vi "update.vi"(0 "OWEN HMI.lvclass":refnum<class "OWEN HMI.lvclass">, 11 "error in":errorcluster) -> (15 "error out":errorcluster)   [LabVIEW 2019, in "OWEN HMI.lvclass"]
uses:
  OWEN HMI.lvclass
  Bit.ctl
  Words.ctl
  19f3744f-72bc-4c39-aaca-5bdf827a74e4.vi
  b80abefe-0104-4203-839a-19dc6cb4a819.vi
  Global - Data.vi
panel:
  in  "stop":bool
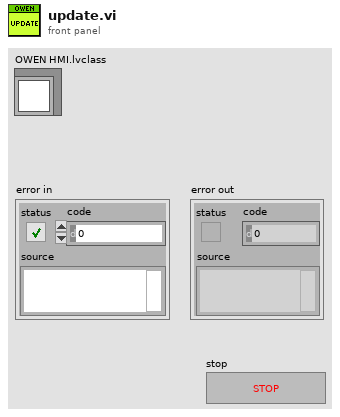
[diagram p1: front panel]
types:
  T1 = typedef "OWEN HMI.lvclass/Bit.ctl" = enum16{"0 - Pump CC", "1 - Pump SO", "2 - Alarm", "3 - Warning", "4 - DUT", "5 - CHMBR"}
  T2 = typedef "OWEN HMI.lvclass/Words.ctl" = enum16{"0 - Bits", "1 - Level CC", "2 - Temp CC", "3 - Level SO", "4 - Temp SO"}
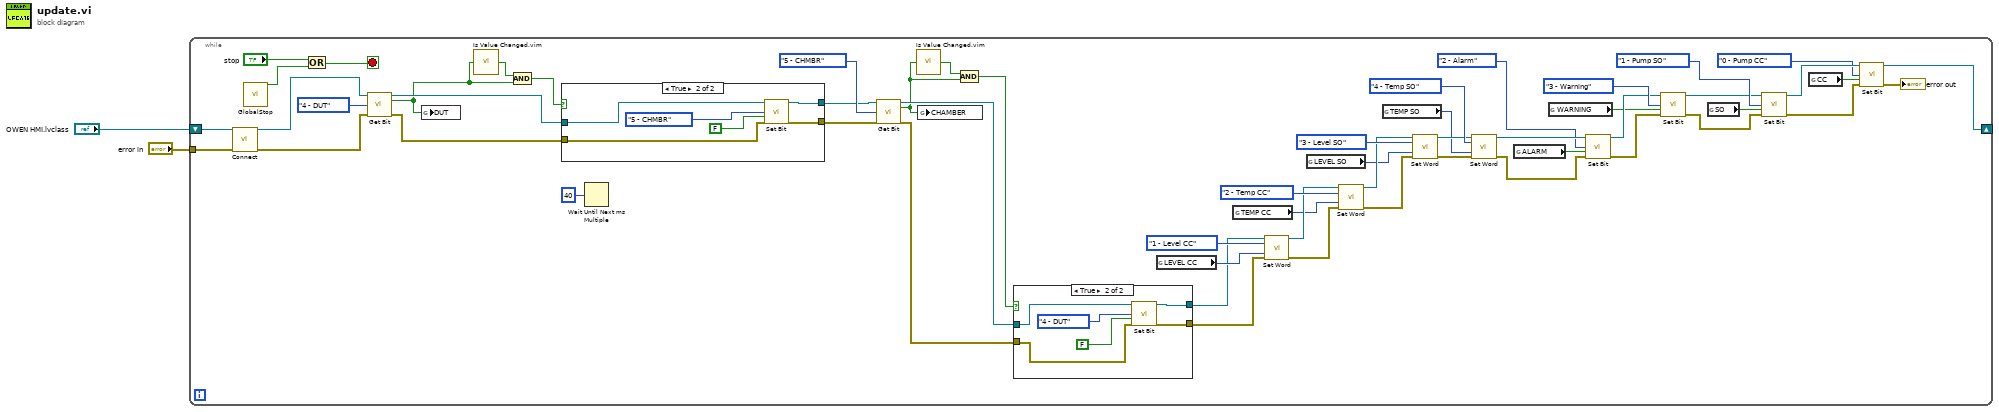
[diagram p0: block diagram]
diagram:
  n1 = while {
    tunnel: "error in" -> [w58]
    shift-right: [w6] -> _
    shift-left: "OWEN HMI.lvclass" -> [w30]
    stop <- w4 stop-if-true
    n2 = call "Connect.vi"("OWEN HMI in"=w30, "error in (no error)"=w58) -> ("OWEN HMI out"=w57:refnum<class "OWEN HMI.lvclass">, "error out"=w56:errorcluster)  [unwired: 12 in]
    n3 = call "GlobalStop.vi"() -> ("Stop"=w3:bool)  [unwired: 15 in]
    n4 = Or(x="stop", y=w3) -> (x .or. y?=w4:bool)
    n5 = call "Get Bit.vi"("OWEN HMI in"=w57, "bit"=Bit."4 - DUT", "error in (no error)"=w56) -> ("OWEN HMI out"=w55:refnum<class "OWEN HMI.lvclass">, "value"=w22:bool, "error out"=w54:errorcluster)  [unwired: 10 in]
    n6 = global write "Global - Data.vi" "DUT"(w22) -> ()
    n7 = call "Is Value Changed.vim"("value"=w22) -> ("changed or first call?"=w21:bool)
    n8 = And(x=w21, y=w22) -> (x .and. y?=w52:bool)
    n9 = case shown="True" w52 {
      tunnel: w55 -> [w68 w74]
      tunnel: w54 -> [w67 w73]
      tunnel: [w68 w71] -> w20
      tunnel: [w67 w70] -> w19
      frame False {
      }
      frame True {
        n10 = call "Set Bit.vi"("OWEN HMI in"=w74, "bit"=Bit."5 - CHMBR", "value"=FALSE, "error in (no error)"=w73) -> ("OWEN HMI out"=w71:refnum<class "OWEN HMI.lvclass">, "error out"=w70:errorcluster)  [unwired: 10 in]
      }
    }
    n11 = Wait Until Next ms Multiple(millisecond multiple=u32 40 ("milliseconds to wait")) -> ()  [unwired: 1 out]
    n12 = call "Get Bit.vi"("OWEN HMI in"=w20, "bit"=Bit."5 - CHMBR", "error in (no error)"=w19) -> ("OWEN HMI out"=w49:refnum<class "OWEN HMI.lvclass">, "value"=w16:bool, "error out"=w50:errorcluster)  [unwired: 10 in]
    n13 = call "Is Value Changed.vim"("value"=w16) -> ("changed or first call?"=w17:bool)
    n14 = global write "Global - Data.vi" "CHAMBER"(w16) -> ()
    n15 = And(x=w17, y=w16) -> (x .and. y?=w51:bool)
    n16 = case shown="True" w51 {
      tunnel: w49 -> [w60 w66]
      tunnel: w50 -> [w59 w65]
      tunnel: [w60 w63] -> w18
      tunnel: [w59 w62] -> w15
      frame False {
      }
      frame True {
        n17 = call "Set Bit.vi"("OWEN HMI in"=w66, "bit"=Bit."4 - DUT", "value"=FALSE, "error in (no error)"=w65) -> ("OWEN HMI out"=w63:refnum<class "OWEN HMI.lvclass">, "error out"=w62:errorcluster)  [unwired: 10 in]
      }
    }
    n18 = global read "Global - Data.vi" "LEVEL CC"() -> (w24:i16)
    n19 = global read "Global - Data.vi" "TEMP CC"() -> (w25:i16)
    n20 = call "Set Word.vi"("OWEN HMI in"=w18, "address"=Words."1 - Level CC", "value"=w24, "error in (no error)"=w15) -> ("OWEN HMI out"=w46:refnum<class "OWEN HMI.lvclass">, "error out"=w45:errorcluster)  [unwired: 10 in]
    n21 = global read "Global - Data.vi" "LEVEL SO"() -> (w26:i16)
    n22 = call "Set Word.vi"("OWEN HMI in"=w46, "address"=Words."2 - Temp CC", "value"=w25, "error in (no error)"=w45) -> ("OWEN HMI out"=w43:refnum<class "OWEN HMI.lvclass">, "error out"=w42:errorcluster)  [unwired: 10 in]
    n23 = global read "Global - Data.vi" "TEMP SO"() -> (w27:i16)
    n24 = call "Set Word.vi"("OWEN HMI in"=w43, "address"=Words."3 - Level SO", "value"=w26, "error in (no error)"=w42) -> ("OWEN HMI out"=w40:refnum<class "OWEN HMI.lvclass">, "error out"=w39:errorcluster)  [unwired: 10 in]
    n25 = call "Set Word.vi"("OWEN HMI in"=w40, "address"=Words."4 - Temp SO", "value"=w27, "error in (no error)"=w39) -> ("OWEN HMI out"=w38:refnum<class "OWEN HMI.lvclass">, "error out"=w37:errorcluster)  [unwired: 10 in]
    n26 = global read "Global - Data.vi" "ALARM"() -> (w29:bool)
    n27 = global read "Global - Data.vi" "WARNING"() -> (w28:bool)
    n28 = call "Set Bit.vi"("OWEN HMI in"=w38, "bit"=Bit."2 - Alarm", "value"=w29, "error in (no error)"=w37) -> ("OWEN HMI out"=w34:refnum<class "OWEN HMI.lvclass">, "error out"=w33:errorcluster)  [unwired: 10 in]
    n29 = call "Set Bit.vi"("OWEN HMI in"=w34, "bit"=Bit."3 - Warning", "value"=w28, "error in (no error)"=w33) -> ("OWEN HMI out"=w7:refnum<class "OWEN HMI.lvclass">, "error out"=w8:errorcluster)  [unwired: 10 in]
    n30 = global read "Global - Data.vi" "SO"() -> (w13:bool)
    n31 = call "Set Bit.vi"("OWEN HMI in"=w7, "bit"=Bit."1 - Pump SO", "value"=w13, "error in (no error)"=w8) -> ("OWEN HMI out"=w11:refnum<class "OWEN HMI.lvclass">, "error out"=w12:errorcluster)  [unwired: 10 in]
    n32 = global read "Global - Data.vi" "CC"() -> (w14:bool)
    n33 = call "Set Bit.vi"("OWEN HMI in"=w11, "bit"=Bit."0 - Pump CC", "value"=w14, "error in (no error)"=w12) -> ("OWEN HMI out"=w6:refnum<class "OWEN HMI.lvclass">, "error out"=→"error out":errorcluster)  [unwired: 10 in]
  }
